vi "总磷启动(子VI).vi"(11 "参数":T2 {"站号" items=["总磷"=1, "总氮"=2, "氨氮"=3]}) -> (0 "error out":T1={"status"=FALSE, "代码"=4, "source"=""} caption="错误输出" {"代码" items=["执行成功"=1, "执行失败，但不知道原因"=2, "命令请求条件错误"=3, "通讯超时"=4, "系统繁忙不能执行"=5, "系统故障"=6, "没有数据"=100]})   [LabVIEW 2016]
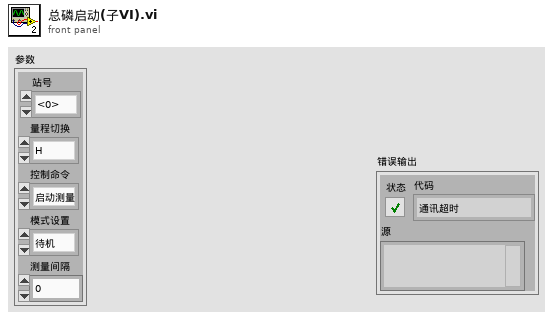
[diagram p1: front panel]
types:
  T1 = cluster{"status":bool, "代码":u16, "source":string}
  T2 = cluster{"站号":u16, "量程切换":enum32{"H", "L", "AUTO"}, "控制命令":enum16{"启动测量", "标样核查", "零点核查", "跨度核查", "空白测试", "平行样测试", "加标回收", "空白校准", "标样校准", "初始化（清洗）", "停止测试", "仪器重启", "校时", "模式设置", "测量间隔设置"}, "模式设置":enum16{"待机", "连续模式", "周期模式", "定点模式", "受控模式", "手动模式"}, "测量间隔":u16}
  T3 = enum16{"空闲", "水样测试", "标样核查", "零点核查", "跨度核查", "空白测试", "平行样测试", "加标回收", "空白校准", "标样校准", "初始化（清洗）"}
  T4 = cluster{"系统时间":timestamp, "工作状态":enum16{"空闲", "水样测试", "标样核查", "零点核查", "跨度核查", "空白测试", "平行样测试", "加标回收", "空白校准", "标样校准", "初始化（清洗）"}, "测量模式":enum16{"待机", "连续模式", "周期模式", "定点模式", "受控模式", "手动模式"}, "告警代码":u16, "故障代码":u16, "日志代码":u16, "软件版本":u16, "F0":sgl, "F1":sgl, "F2":sgl, "F3":sgl, "T":sgl, "H":sgl, "id":u16, "flowid":u16, "量程":u16, "总磷控温温度1":sgl, "营养盐控温温度2":sgl, "ADC":sgl}
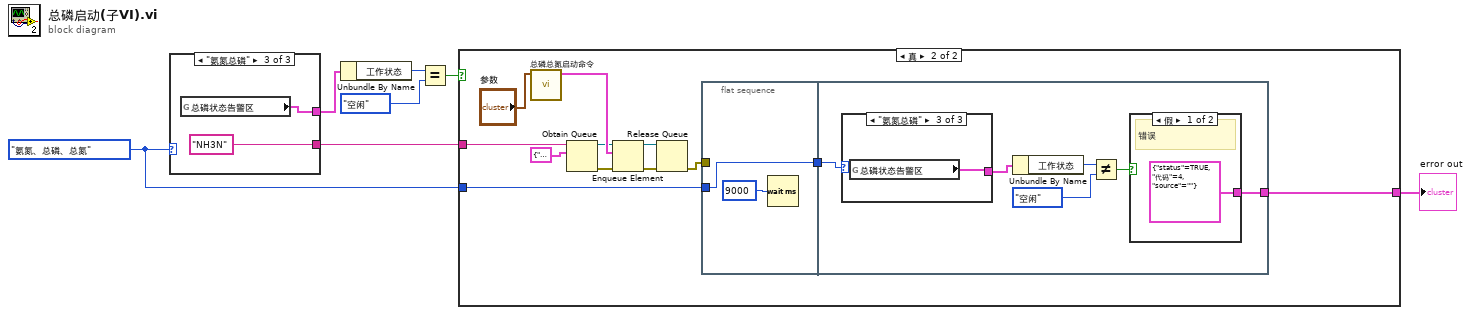
[diagram p0: block diagram]
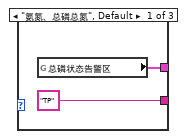
[diagram p2: hidden frame]
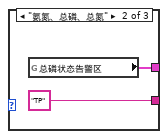
[diagram p3: hidden frame]
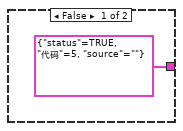
[diagram p4: hidden frame]
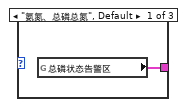
[diagram p5: hidden frame]
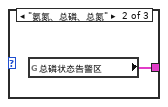
[diagram p6: hidden frame]
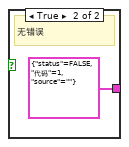
[diagram p7: hidden frame]
diagram:
  w1 = enum16{"氨氮、总磷总氮", "氨氮总磷", "氨氮、总磷、总氮"}."氨氮、总磷、总氮" ("营养盐类型")
  n1 = case shown="\"氨氮总磷\"" w1 {
    tunnel: [w9 w11 w12] -> w4
    tunnel: ["TP" ("名称（未命名）") "TP" ("名称（未命名）") "NH3N" ("名称（未命名）")] -> w2
    frame "氨氮、总磷总氮", Default {
      n2 = global read "VAR总磷总氮全局变量.vi" "总磷状态告警区"() -> (w9:T4)
    }
    frame "氨氮、总磷、总氮" {
      n3 = global read "VAR总磷总氮全局变量.vi" "总磷状态告警区"() -> (w11:T4)
    }
    frame "氨氮总磷" {
      n4 = global read "VAR总磷总氮全局变量.vi" "总磷状态告警区"() -> (w12:T4)
    }
  }
  n5 = Unbundle By Name(w4) -> ("工作状态"=w7:T3)
  n6 = Equal?(x=w7, y=T3."空闲") -> (x = y?=w5:bool)
  n7 = case shown="真" w5 {
    tunnel: [T1 {"status"=TRUE, "代码"=5, "source"=""} ("error out") w18] -> w3
    tunnel: w2 -> [_ w17]
    tunnel: w1 -> [_ w15]
    frame False {
    }
    frame True {
      n8 = call "总磷总氮启动命令.vi"("参数"="参数") -> ("启动命令"=w26:cluster{"命令":string, "data":variant})  [unwired: 10 in]
      n9 = Obtain Queue(name (unnamed)=w17, element data type=cluster{"命令":string, "data":variant} {"命令"="", "data"=variant}) -> (queue out=w23:refnum<queue>, error out=w24:errorcluster)  [unwired: 3 in, 1 out]
      n10 = Enqueue Element(queue=w23, element=w26, error in (no error)=w24) -> (queue out=w21:refnum<queue>, error out=w20:errorcluster)  [unwired: 1 in, 1 out]
      n11 = Release Queue(queue=w21, error in (no error)=w20) -> (error out=w19:errorcluster)  [unwired: 1 in, 2 out]
      n12 = flat-sequence {
        tunnel: w19 -> [_]
        tunnel: [w27] -> w16
        tunnel: w15 -> [w27]
        tunnel: [w34] -> w18
        tunnel: w16 -> [w30]
        frame #0 {
          n13 = Wait (ms)(milliseconds to wait=u32 9000 ("等待时间（毫秒）")) -> ()  [unwired: 1 out]
        }
        frame #1 {
          n14 = case shown="\"氨氮总磷\"" w30 {
            tunnel: [w35 w36 w37] -> w29
            frame "氨氮、总磷总氮", Default {
              n15 = global read "VAR总磷总氮全局变量.vi" "总磷状态告警区"() -> (w35:T4)
            }
            frame "氨氮、总磷、总氮" {
              n16 = global read "VAR总磷总氮全局变量.vi" "总磷状态告警区"() -> (w36:T4)
            }
            frame "氨氮总磷" {
              n17 = global read "VAR总磷总氮全局变量.vi" "总磷状态告警区"() -> (w37:T4)
            }
          }
          n18 = Unbundle By Name(w29) -> ("工作状态"=w32:T3)
          n19 = Not Equal?(x=w32, y=T3."空闲") -> (x != y?=w31:bool)
          n20 = case shown="假" w31 {
            tunnel: [T1 {"status"=TRUE, "代码"=4, "source"=""} ("error out") T1 {"status"=FALSE, "代码"=1, "source"=""} ("error out")] -> w34
            frame False {
              # "错误"
            }
            frame True {
              # "无错误"
            }
          }
        }
      }
    }
  }
  "error out" <- w3
